vi "Gen_Fahr.vi"() -> (0 "Temp (F)":dbl(slide) scale=0.0..110.0)   [LabVIEW 2024]
doc: "Questo blocco simula una temperatura in gradi Fahrenheit."
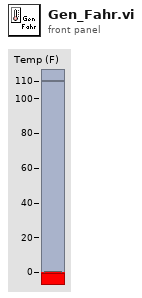
[diagram p1: front panel]
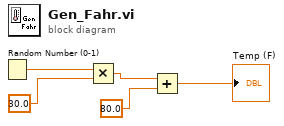
[diagram p0: block diagram]
diagram:
  n1 = Random Number (0-1)() -> (number: 0 to 1=w5:dbl)
  n2 = Multiply(x=w5, y=30.0) -> (x*y=w3:dbl)
  n3 = Add(x=w3, y=80.0) -> (x+y=→"Temp (F)":dbl)
